vi "Select Image File.vi"(8 "error in (no error)":errorcluster caption="错误输入（无错误）", 11 "文件路径输入控件":path) -> (0 "error out":errorcluster caption="错误输出", 3 "image data":T1)   [LabVIEW 2011]
uses:
  <vilib>/picture/picture.llb/imagedata.ctl
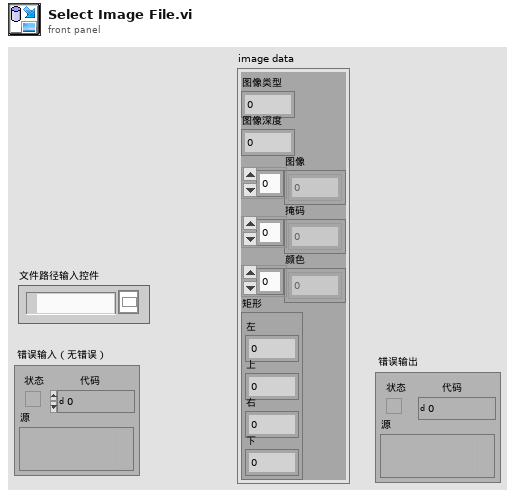
[diagram p1: front panel]
types:
  T1 = typedef "imagedata.ctl" = cluster{"image type":i32, "image depth":i32, "image":u8[], "mask":u8[], "colors":u32[], "Rectangle":cluster{"left":i16, "top":i16, "right":i16, "bottom":i16}}
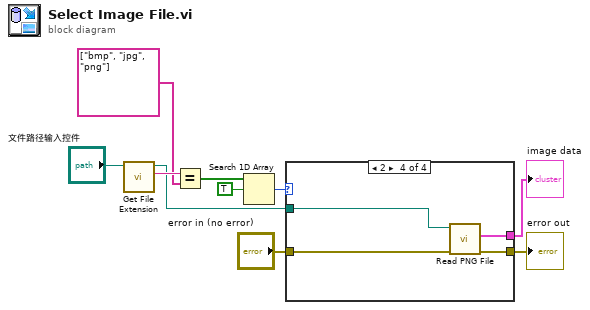
[diagram p0: block diagram]
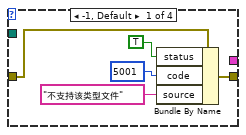
[diagram p2: hidden frame]
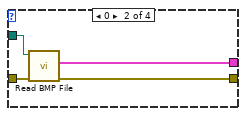
[diagram p3: hidden frame]
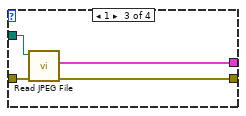
[diagram p4: hidden frame]
diagram:
  n1 = call <vilib>:"Get File Extension.vi"("file"="文件路径输入控件") -> ("lowercase file extension"=w9:string, "dup file"=w4:path)  [unwired: 7 in, 2 out]
  n2 = Equal?(x=w9, y=string[] ["bmp", "jpg", "png"]) -> (x = y?=w7:bool[])
  n3 = Search 1D Array(1D array=w7, element=TRUE ("元素")) -> (index of element=w5:i32)  [unwired: 1 in]
  n4 = case shown="2" w5 {
    tunnel: w4 -> [_ w19 w23 w27]
    tunnel: "error in (no error)" -> [w15 w18 w22 w26]
    tunnel: [w11 w17 w21 w25] -> w2
    tunnel: [_ w16 w20 w24] -> w1
    frame -1, Default {
      n5 = Bundle By Name(cluster=w15, "status"=TRUE, "code"=5001, "source"="不支持该类型文件") -> (w11:errorcluster)
    }
    frame 0 {
      n6 = call <vilib>:"Read BMP File.vi"("error in (no error)"=w18, "path to BMP file"=w19) -> ("error out"=w17:errorcluster, "image data"=w16:T1)  [unwired: 7 in, 1 out]
    }
    frame 1 {
      n7 = call <vilib>:"Read JPEG File.vi"("error in (no error)"=w22, "path to JPEG file"=w23) -> ("error out"=w21:errorcluster, "image data"=w20:T1)  [unwired: 7 in, 1 out]
    }
    frame 2 {
      n8 = call <vilib>:"Read PNG File.vi"("error in (no error)"=w26, "path to PNG file"=w27) -> ("error out"=w25:errorcluster, "image data"=w24:T1)  [unwired: 7 in, 1 out]
    }
  }
  "error out" <- w2
  "image data" <- w1
